vi "GetTypeMap.vi"(8 "error in (no error)":errorcluster, 11 "object in":refnum<class>) -> (0 "error out":errorcluster, 1 "found":bool, 2 "TypeMap":refnum<class "TypeMap.lvclass">, 3 "object out":refnum<class>)   [LabVIEW 2020, in "ORM_API.lvlib"]
uses:
  ORM_API.lvlib
  <vilib>/Viviota/shared/ORM.lvlibp/ORM/TypeMap/TypeMap.lvclass
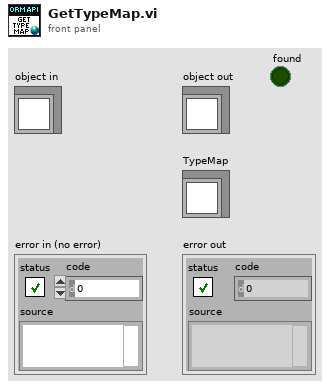
[diagram p1: front panel]
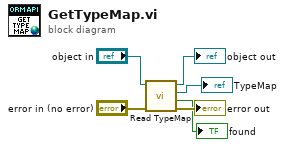
[diagram p0: block diagram]
diagram:
  n1 = call <vilib>:"Read TypeMap.vi"("error in (no error)"="error in (no error)", "object in"="object in") -> ("error out"=→"error out":errorcluster, "found/replaced?"=→"found":bool, "TypeMap in"=→"TypeMap":refnum<class "TypeMap.lvclass">, "object out"=→"object out":refnum<class>)  [unwired: 6 in]
